vi "ReadMaxDataInputSize.vi"(8 "Error In":errorcluster) -> (0 "Error Out":errorcluster, 1 "Max Data Input Size":i32=-1)   [LabVIEW 2018, in "TracerLibrary.lvlib" / "Tracer.lvclass"]
uses:
  Tracer.lvclass
  protected/Tracer_ClassAttributes.vi
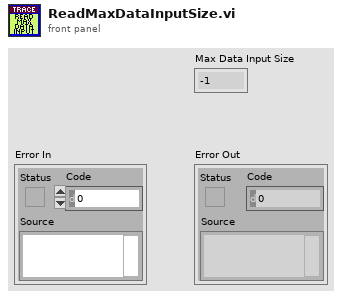
[diagram p1: front panel]
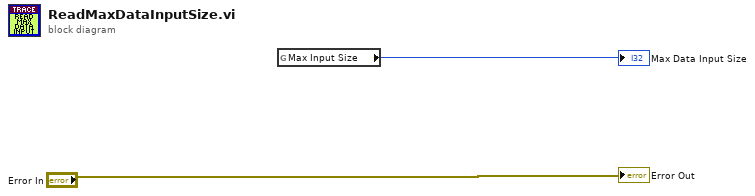
[diagram p0: block diagram]
diagram:
  n1 = global read "Tracer_ClassAttributes.vi" "Max Input Size"() -> (→"Max Data Input Size":i32)
  "Error Out" <- "Error In"
